vi "save design values.vi"(8 "error in":errorcluster, 9 "User Information":T1 {"Country" items=["Afghanistan", "Aland Islands", "Albania", "Algeria", "American Samoa", "Andorra", "Angola", "Anguilla", "Antarctica", "Antigua And Barbuda", "Argentina", "Armenia", "Aruba", "Australia", "Austria", "Azerbaijan", "Bahamas", "Bahrain", "Bangladesh", "Barbados", "Belarus", "Belgium", "Belize", "Benin", "Bermuda", "Bhutan", "Bolivia", "Bosnia And Herzegovina", "Botswana", "Bouvet Island", "Brazil", "British Indian Ocean Territory", "Brunei Darussalam", "Bulgaria", "Burkina Faso", "Burundi", "Cambodia", "Cameroon", "Canada", "Cape Verde", "Cayman Islands", "Central African Republic", "Chad", "Chile", "China", "Christmas Island", "Cocos (Keeling) Islands", "Colombia", "Comoros", "Congo", "Congo, The Democratic Republic Of The", "Cook Islands", "Costa Rica", "Cote D'Ivoire", "Croatia", "Cuba", "Cyprus", "Czech Republic", "Denmark", "Djibouti", "Dominica", "Dominican Republic", "Ecuador", "Egypt", "El Salvador", "Equatorial Guinea", "Eritrea", "Estonia", "Ethiopia", "Falkland Islands (Malvinas)", "Faroe Islands", "Fiji", "Finland", "France", "French Guiana", "French Polynesia", "French Southern Territories", "Gabon", "Gambia", "Georgia", "Germany", "Ghana", "Gibraltar", "Greece", "Greenland", "Grenada", "Guadeloupe", "Guam", "Guatemala", "Guernsey", "Guinea", "Guinea-Bissau", "Guyana", "Haiti", "Heard Island And Mcdonald Islands", "Holy See (Vatican City State)", "Honduras", "Hong Kong", "Hungary", "Iceland", "India", "Indonesia", "Iran, Islamic Republic Of", "Iraq", "Ireland", "Isle Of Man", "Israel", "Italy", "Jamaica", "Japan", "Jersey", "Jordan", "Kazakhstan", "Kenya", "Kiribati", "Korea, Democratic People'S Republic Of", "Korea, Republic Of", "Kuwait", "Kyrgyzstan", "Lao People'S Democratic Republic", "Latvia", "Lebanon", "Lesotho", "Liberia", "Libyan Arab Jamahiriya", "Liechtenstein", "Lithuania", "Luxembourg", "Macao", "Macedonia, The Former Yugoslav Republic Of", "Madagascar", "Malawi", "Malaysia", "Maldives", "Mali", "Malta", "Marshall Islands", "Martinique", "Mauritania", "Mauritius", "Mayotte", "Mexico", "Micronesia, Federated States Of", "Moldova, Republic Of", "Monaco", "Mongolia", "Montserrat", "Morocco", "Mozambique", "Myanmar", "Namibia", "Nauru", "Nepal", "Netherlands", "Netherlands Antilles", "New Caledonia", "New Zealand", "Nicaragua", "Niger", "Nigeria", "Niue", "Norfolk Island", "Northern Mariana Islands", "Norway", "Oman", "Pakistan", "Palau", "Palestinian Territory, Occupied", "Panama", "Papua New Guinea", "Paraguay", "Peru", "Philippines", "Pitcairn", "Poland", "Portugal", "Puerto Rico", "Qatar", "Reunion", "Romania", "Russian Federation", "Rwanda", "Saint Helena", "Saint Kitts And Nevis", "Saint Lucia", "Saint Pierre And Miquelon", "Saint Vincent And The Grenadines", "Samoa", "San Marino", "Sao Tome And Principe", "Saudi Arabia", "Senegal", "Serbia And Montenegro", "Seychelles", "Sierra Leone", "Singapore", "Slovakia", "Slovenia", "Solomon Islands", "Somalia", "South Africa", "South Georgia And The South Sandwich Islands", "Spain", "Sri Lanka", "Sudan", "Suriname", "Svalbard And Jan Mayen", "Swaziland", "Sweden", "Switzerland", "Syrian Arab Republic", "Taiwan, Province Of China", "Tajikistan", "Tanzania, United Republic Of", "Thailand", "Timor-Leste", "Togo", "Tokelau", "Tonga", "Trinidad And Tobago", "Tunisia", "Turkey", "Turkmenistan", "Turks And Caicos Islands", "Tuvalu", "Uganda", "Ukraine", "United Arab Emirates", "United Kingdom", "United States", "United States Minor Outlying Islands", "Uruguay", "Uzbekistan", "Vanuatu", "Venezuela", "Viet Nam", "Virgin Islands, British", "Virgin Islands, U.S.", "Wallis And Futuna", "Western Sahara", "Yemen", "Zambia", "Zimbabwe", "(Not Specified)"]}, 10 "MathCAD results":T3, 11 "Project Folder":path) -> (0 "error out":errorcluster)   [LabVIEW 2015, in "AguaClara Library.lvlib"]
uses:
  AguaClara Library.lvlib
  User Information.ctl
  MathCAD results ref.ctl
  Country Ring.ctl
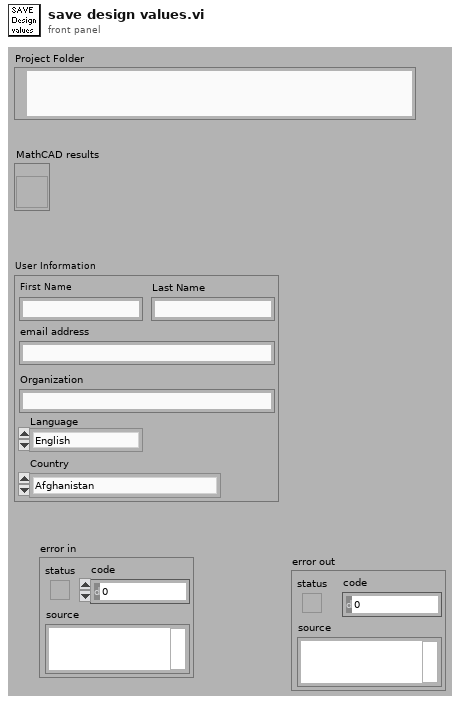
[diagram p1: front panel]
types:
  T1 = typedef "AguaClara Library.lvlib/User Information.ctl" = cluster{"First Name":string, "Last Name":string, "Email Address":string, "Organization":string, "Language":enum16{"English", "Español", "French"}, "Country":T2}
  T2 = typedef "Country Ring.ctl" = u16
  T3 = typedef "MathCAD results ref.ctl" = refnum<vi>
  T4 = enum16{"open", "replace", "create", "open or create", "replace or create", "replace or create with confirmation"}
  T5 = cluster{"Label.Text":string, "Caption.Text":string[], "Control Type":u32, "Numeric":dbl, "Array":dbl[], "status":bool, "Outputs":bool[], "Str Array":string[], "String":string}[]
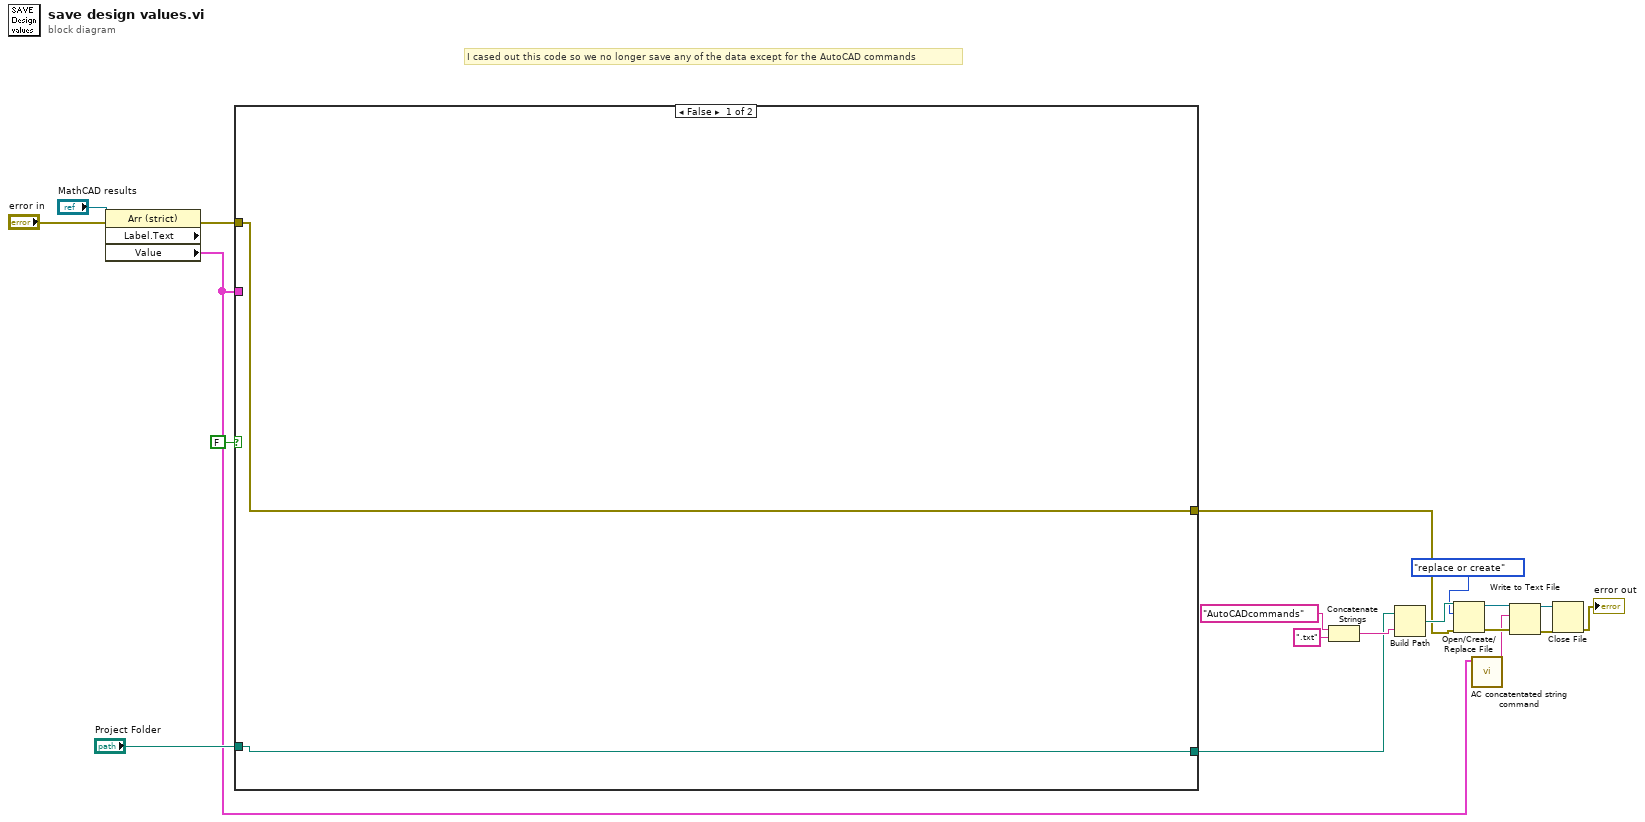
[diagram p0: block diagram]
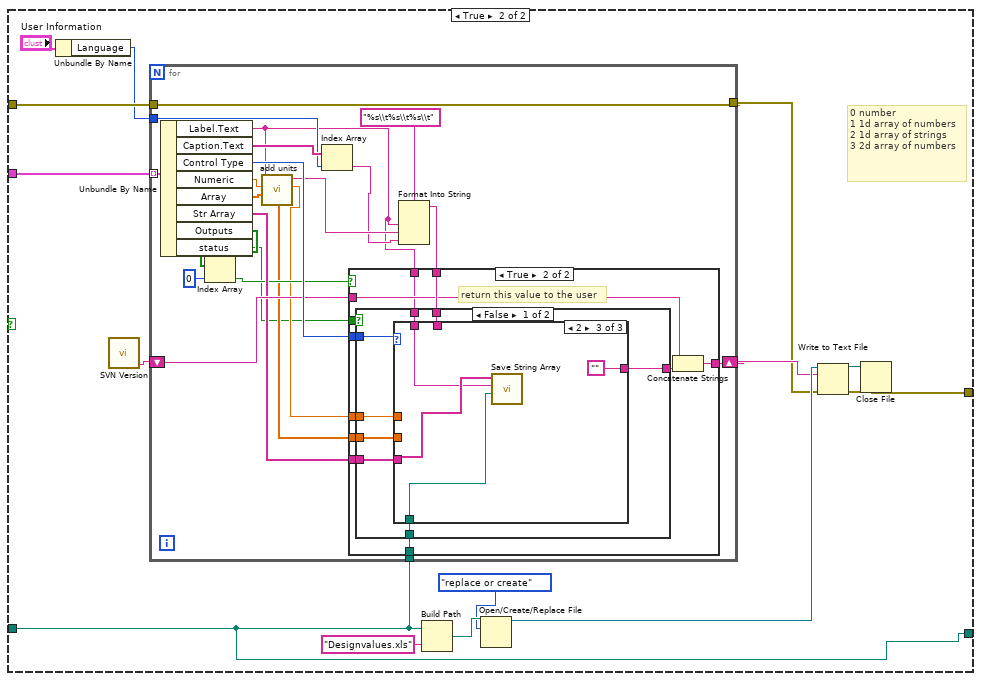
[diagram p2: hidden frame]
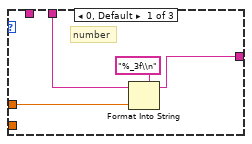
[diagram p4: hidden frame]
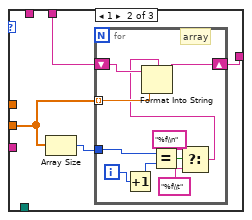
[diagram p5: hidden frame]
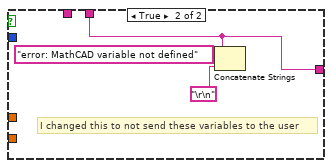
[diagram p6: hidden frame]
diagram:
  # "I cased out this code so we no longer save any of the data except for the AutoCAD commands"
  n1 = property class="Arr (strict)" props=["Label", "Text", "Value"](reference="MathCAD results", error in="error in") -> (error out=w17:errorcluster, "Value"=w6:T5)  [unwired: 2 out]
  n2 = case shown="False" FALSE {
    tunnel: w17 -> [w21 w28]
    tunnel: "Project Folder" -> [w20 w22]
    tunnel: w6 -> [_ w24]
    tunnel: [w21 w23] -> w5
    tunnel: [w20 w22] -> w1
    frame False {
    }
    frame True {
      # "0\tnumber\n1\t1d array of numbers\n2\t1d array of strings\n3\t2d array of numbers"
      n3 = Unbundle By Name("User Information") -> ("Language"=w26:enum16{"English", "Español", "French"})
      n4 = call "SVN Version.vi"() -> ("Version string"=w25:string)  [unwired: 7 in, 4 out]
      n5 = for {
        tunnel: w28 -> [w56]
        tunnel: [w56] -> w29
        shift-right: [w48] -> w33
        shift-left: w25 -> [w49]
        tunnel: w24 -> [w58] mode=indexing
        tunnel: w26 -> [w54]
        tunnel: w22 -> [w37]
        n6 = Unbundle By Name(w58) -> ("Label.Text"=w38:string, "Caption.Text"=w55:string[], "Control Type"=w57:u32, "Numeric"=w42:dbl, "Array"=w43:dbl[], "Str Array"=w47:string[], "Outputs"=w46:bool[], "status"=w39:bool)
        n7 = Index Array(array=w46, index=0) -> (element=w44:bool)
        n8 = call "add units.vi"("Array"=w43, "Numeric"=w42, "Label Text"=w38) -> ("Converted Array"=w41:dbl[], "Converted Numeric"=w40:dbl, "unit in brackets"=w53:string)  [unwired: 4 in, 2 out]
        n9 = Index Array(array=w55, index=w54) -> (element=w52:string)
        n10 = Format Into String(format string="%s\\t%s\\t%s\\t", w38, w53, w52) -> (resulting string=w50:string)  [unwired: 2 in, 1 out]
        n11 = case shown="True" w44 {
          tunnel: w57 -> [_ w70]
          tunnel: w40 -> [_ w69]
          tunnel: w41 -> [_ w68]
          tunnel: w50 -> [_ w67]
          tunnel: w49 -> [w59 w65]
          tunnel: [w59 w64] -> w48
          tunnel: w47 -> [_ w63]
          tunnel: w39 -> [_ w62]
          tunnel: w38 -> [_ w61]
          tunnel: w37 -> [_ w60]
          frame False {
            # "don't return this value to the user"
          }
          frame True {
            # "return this value to the user"
            n12 = case shown="False" w62 {
              tunnel: w70 -> [w78 _]
              tunnel: w69 -> [w77 _]
              tunnel: w68 -> [w76 _]
              tunnel: w67 -> [w75 w101]
              tunnel: [w74 w101] -> w66
              tunnel: w63 -> [w73 _]
              tunnel: w61 -> [w72 _]
              tunnel: w60 -> [w71 _]
              frame False {
                n13 = case shown="2" w78 {
                  tunnel: [w79 w86 ""] -> w74
                  tunnel: w77 -> [w80 _ _]
                  tunnel: w76 -> [_ w84 _]
                  tunnel: w75 -> [w81 w83 _]
                  tunnel: w73 -> [_ _ w99]
                  tunnel: w72 -> [_ _ w98]
                  tunnel: w71 -> [_ _ w97]
                  frame 0, Default {
                    # "number"
                    n14 = Format Into String(format string="%_3f\\n", initial string=w81, w80) -> (resulting string=w79:string)  [unwired: 1 in, 1 out]
                  }
                  frame 1 {
                    n15 = Array Size(array=w84) -> (size(s)=w85:i32)
                    n16 = for {
                      shift-right: [w95] -> w86
                      shift-left: w83 -> [w96]
                      tunnel: w84 -> [w94] mode=indexing
                      tunnel: w85 -> [w88]
                      i -> [w93]
                      # "array"
                      n17 = Increment(x=w93) -> (x+1=w87:i32)
                      n18 = Equal?(x=w88, y=w87) -> (x = y?=w92:bool)
                      n19 = Select(t="%f\\n" ("format string"), s=w92, f="%f\\t" ("format string")) -> (s? t:f=w89:string)
                      n20 = Format Into String(format string=w89, initial string=w96, w94) -> (resulting string=w95:string)  [unwired: 1 in, 1 out]
                    }
                  }
                  frame 2 {
                    n21 = call "Save String Array.vi"("Project Folder"=w97, "Label"=w98, "Str Array"=w99) -> ()  [unwired: 8 in, 1 out]
                  }
                }
              }
              frame True {
                # "I changed this to not send these variables to the user"
                n22 = Concatenate Strings(w101, "error: MathCAD variable not defined" ("string"), "\r\n") -> ()  [unwired: 1 out]
              }
            }
            n23 = Concatenate Strings(w65, w66) -> (w64:string)
          }
        }
      }
      n24 = Build Path(base path=w22, name or relative path="Designvalues.xls") -> (appended path=w36:path)
      n25 = Open/Create/Replace File(file path (use dialog)=w36, operation (0:open)=T4."replace or create") -> (refnum out=w34:refnum<file>)  [unwired: 4 in, 2 out]
      n26 = Write to Text File(file (use dialog)=w34, text=w33, error in=w29) -> (refnum out=w31:refnum<file>, error out=w32:errorcluster)  [unwired: 1 in, 1 out]
      n27 = Close File(refnum=w31, error in=w32) -> (error out=w23:errorcluster)  [unwired: 1 out]
    }
  }
  n28 = Concatenate Strings("AutoCADcommands" ("string"), ".txt" ("string")) -> (w11:string)
  n29 = Build Path(base path=w1, name or relative path=w11) -> (appended path=w16:path)
  n30 = Open/Create/Replace File(file path (use dialog)=w16, error in=w5, operation (0:open)=T4."replace or create") -> (refnum out=w10:refnum<file>, error out=w9:errorcluster)  [unwired: 3 in, 1 out]
  n31 = call "AC concatentated string command.vi"("MathCAD results"=w6) -> ("AC concatenated string"=w7:string)  [unwired: 10 in]
  n32 = Write to Text File(file (use dialog)=w10, text=w7, error in=w9) -> (refnum out=w13:refnum<file>, error out=w14:errorcluster)  [unwired: 1 in, 1 out]
  n33 = Close File(refnum=w13, error in=w14) -> (error out=→"error out":errorcluster)  [unwired: 1 out]
